vi "globState.vi"() -> ()   [LabVIEW 2023]
panel:
  in  "State":T1(ring)
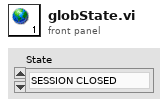
[diagram p1: front panel]
types:
  T1 = enum16{"SESSION CLOSED", "WAIT", "TEST WAIT", "TEST IN PROGESS", "BATCH IN PROGRESS"}
diagram:
